vi "Initialize Instrument.vi"(8 "error in (no error)":errorcluster, 10 "Reset":bool, 11 "PM-EMP in":refnum<class "PM-EMP.lvclass">) -> (0 "error out":errorcluster, 3 "PM-EMP out":refnum<class "PM-EMP.lvclass">)   [LabVIEW 2020, in "PM-EMP.lvclass"]
uses:
  PM-EMP.lvclass
  C:/Sandbox/RF Bench/Source Code/WiSpry Test Framework/Instruments/Instrument.lvclass
  Instrument.lvclass/Instrument.ctl
  Instrument.lvclass
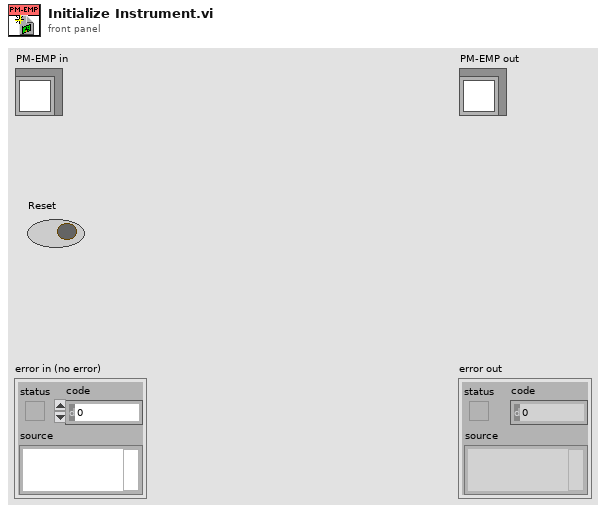
[diagram p1: front panel]
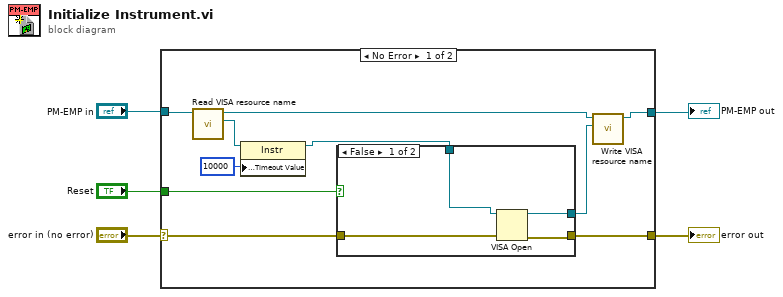
[diagram p0: block diagram]
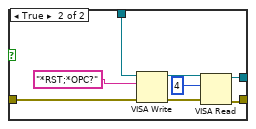
[diagram p2: hidden frame]
diagram:
  n1 = case shown="No Error" "error in (no error)" {
    selector: "error in (no error)" -> [w13 w29]
    tunnel: [w14 w29] -> w4
    tunnel: "PM-EMP in" -> [w15 w28]
    tunnel: [w7 w28] -> w2
    tunnel: "Reset" -> [w12 _]
    frame No Error {
      n2 = call "Read VISA resource name.vi"("Instrument in"=w15) -> ("VISA resource name"=w10:refnum<visa-resource-name>, "Instrument out"=w8:refnum<class "PM-EMP.lvclass">)  [unwired: 9 in]
      n3 = property class="Instr"(reference=w10, "General Settings:Timeout Value"=u32 10000) -> (reference out=w9:refnum<visa-resource-name>)  [unwired: 1 in, 1 out]
      n4 = case shown="False" w12 {
        tunnel: [w19 w22] -> w14
        tunnel: w9 -> [w17 w27]
        tunnel: w13 -> [w16 w26]
        tunnel: [w18 w20] -> w6
        frame False {
          n5 = VISA Open(error in (no error)=w16, VISA resource name=w17) -> (VISA resource name=w18:refnum<visa-resource-name>, error out=w19:errorcluster)  [unwired: 3 in]
        }
        frame True {
          n6 = VISA Write(VISA resource name=w27, write buffer="*RST;*OPC?", error in (no error)=w26) -> (VISA resource name out=w23:refnum<visa-resource-name>, error out=w24:errorcluster)  [unwired: 1 out]
          n7 = VISA Read(VISA resource name=w23, byte count=u32 4, error in (no error)=w24) -> (VISA resource name out=w20:refnum<visa-resource-name>, error out=w22:errorcluster)  [unwired: 2 out]
        }
      }
      n8 = call "Write VISA resource name.vi"("VISA resource name"=w6, "Instrument in"=w8) -> ("Instrument out"=w7:refnum<class "PM-EMP.lvclass">)  [unwired: 9 in]
    }
    frame Error {
    }
  }
  "error out" <- w4
  "PM-EMP out" <- w2
